vi "getJoystickValues.vi"(4 "povType":T1(ring), 6 "Mode":enum16{"Axis", "Button", "POV"}(ring), 8 "error in (no error)":errorcluster, 9 "axisType":T2(ring), 10 "buttonType":T3(ring), 11 "JoystickDevRef":T4) -> (0 "error out":errorcluster, 1 "Button Pressed":bool, 2 "Value":dbl, 3 "JoystickDevRef":T4)   [LabVIEW 2016, in "External.lvlib"]
uses:
  External.lvlib
  <vilib>/Rock Robotics/WPI/Joystick/WPI_JoystickDevRef.ctl
  <vilib>/Rock Robotics/WPI/Joystick/WPI_JoystickDeviceEnum.ctl
  Index.vi
  External/axisValue.vi
  External/POV.vi
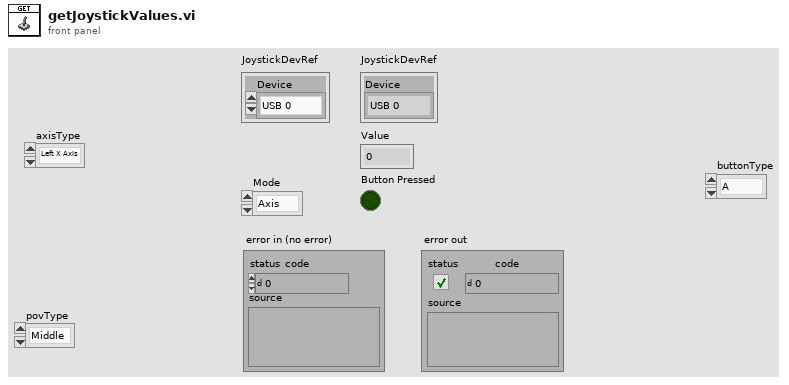
[diagram p1: front panel]
types:
  T1 = enum16{"Middle", "Left", "Left-Down", "Down", "Right-Down", "Right", "Right-Up", "Up", "Left-Up"}
  T2 = enum16{"Left X Axis", "Left Y Axis", "Left Trigger", "Right Trigger", "Right X Axis", "Right Y Axis"}
  T3 = enum16{"A", "B", "X", "Y", "LB", "RB", "Back", "Start", "Left Joystick Pressure Button", "Right Joystick Pressure Button"}
  T4 = typedef "WPI_JoystickDevRef.ctl" = cluster{"Device":T5}
  T5 = typedef "WPI_JoystickDeviceEnum.ctl" = enum16{"USB 0", "USB 1", "USB 2", "USB 3", "USB 4", "USB 5"}
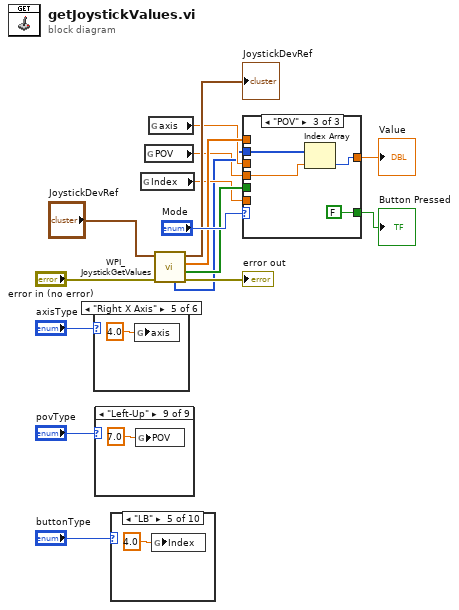
[diagram p0: block diagram]
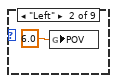
[diagram p3: hidden frame]
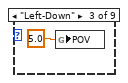
[diagram p4: hidden frame]
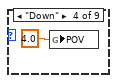
[diagram p5: hidden frame]
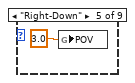
[diagram p6: hidden frame]
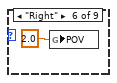
[diagram p7: hidden frame]
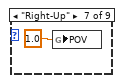
[diagram p8: hidden frame]
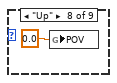
[diagram p9: hidden frame]
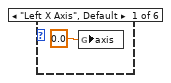
[diagram p10: hidden frame]
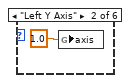
[diagram p11: hidden frame]
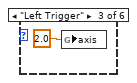
[diagram p12: hidden frame]
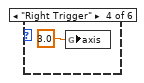
[diagram p13: hidden frame]
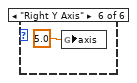
[diagram p14: hidden frame]
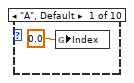
[diagram p15: hidden frame]
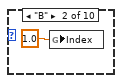
[diagram p16: hidden frame]
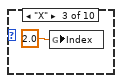
[diagram p17: hidden frame]
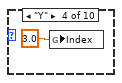
[diagram p18: hidden frame]
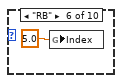
[diagram p19: hidden frame]
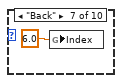
[diagram p20: hidden frame]
diagram:
  n1 = case shown="\"Right X Axis\"" "axisType" {
    frame "Left X Axis", Default {
      n2 = global write "axisValue.vi" "axis"(0.0 ("axis")) -> ()
    }
    frame "Left Y Axis" {
      n3 = global write "axisValue.vi" "axis"(1.0 ("axis")) -> ()
    }
    frame "Left Trigger" {
      n4 = global write "axisValue.vi" "axis"(2.0 ("axis")) -> ()
    }
    frame "Right Trigger" {
      n5 = global write "axisValue.vi" "axis"(3.0 ("axis")) -> ()
    }
    frame "Right X Axis" {
      n6 = global write "axisValue.vi" "axis"(4.0 ("axis")) -> ()
    }
    frame "Right Y Axis" {
      n7 = global write "axisValue.vi" "axis"(5.0 ("axis")) -> ()
    }
  }
  n8 = case shown="\"Left-Up\"" "povType" {
    frame "Middle", Default {
    }
    frame "Left" {
      n9 = global write "POV.vi" "POV"(6.0 ("POV")) -> ()
    }
    frame "Left-Down" {
      n10 = global write "POV.vi" "POV"(5.0 ("POV")) -> ()
    }
    frame "Down" {
      n11 = global write "POV.vi" "POV"(4.0 ("POV")) -> ()
    }
    frame "Right-Down" {
      n12 = global write "POV.vi" "POV"(3.0 ("POV")) -> ()
    }
    frame "Right" {
      n13 = global write "POV.vi" "POV"(2.0 ("POV")) -> ()
    }
    frame "Right-Up" {
      n14 = global write "POV.vi" "POV"(1.0 ("POV")) -> ()
    }
    frame "Up" {
      n15 = global write "POV.vi" "POV"(0.0 ("POV")) -> ()
    }
    frame "Left-Up" {
      n16 = global write "POV.vi" "POV"(7.0 ("POV")) -> ()
    }
  }
  n17 = case shown="\"LB\"" "buttonType" {
    frame "A", Default {
      n18 = global write "Index.vi" "Index"(0.0 ("Index")) -> ()
    }
    frame "B" {
      n19 = global write "Index.vi" "Index"(1.0 ("Index")) -> ()
    }
    frame "X" {
      n20 = global write "Index.vi" "Index"(2.0 ("Index")) -> ()
    }
    frame "Y" {
      n21 = global write "Index.vi" "Index"(3.0 ("Index")) -> ()
    }
    frame "LB" {
      n22 = global write "Index.vi" "Index"(4.0 ("Index")) -> ()
    }
    frame "RB" {
      n23 = global write "Index.vi" "Index"(5.0 ("Index")) -> ()
    }
    frame "Back" {
      n24 = global write "Index.vi" "Index"(6.0 ("Index")) -> ()
    }
    frame "Start" {
      n25 = global write "Index.vi" "Index"(7.0 ("Index")) -> ()
    }
    frame "Left Joystick Pressure Button" {
      n26 = global write "Index.vi" "Index"(8.0 ("Index")) -> ()
    }
    frame "Right Joystick Pressure Button" {
      n27 = global write "Index.vi" "Index"(9.0 ("Index")) -> ()
    }
  }
  n28 = global read "Index.vi" "Index"() -> (w6:dbl)
  n29 = global read "POV.vi" "POV"() -> (w1:dbl)
  n30 = global read "axisValue.vi" "axis"() -> (w5:dbl)
  n31 = call <vilib>:"WPI_JoystickGetValues.vi"("error in (no error)"="error in (no error)", "JoystickDevRef"="JoystickDevRef") -> ("error out"=→"error out":errorcluster, "Buttons"=w7:bool[], "Axes"=w15:dbl[], "JoystickDevRef"=→"JoystickDevRef":T4, "POVs"=w3:i16[])  [unwired: 5 in]
  n32 = case shown="\"POV\"" "Mode" {
    tunnel: w15 -> [w44 _ _]
    tunnel: w7 -> [_ w48 _]
    tunnel: w5 -> [w43 _ _]
    tunnel: [w42 0.0 ("upper limit") w50] -> w13
    tunnel: [FALSE w47 FALSE] -> w12
    tunnel: w6 -> [_ w45 _]
    tunnel: w3 -> [_ _ w52]
    tunnel: w1 -> [_ _ w51]
    frame "Axis", Default {
      n33 = Index Array(array=w44, index=w43) -> (element=w42:dbl)
    }
    frame "Button" {
      n34 = Index Array(array=w48, index=w45) -> (element=w47:bool)
    }
    frame "POV" {
      n35 = Index Array(array=w52, index=w51) -> (element=w50:i16)
    }
  }
  "Value" <- w13
  "Button Pressed" <- w12
